vi "delete PID from configuration.vi"(8 "error in":errorcluster, 10 "PID Loop ID In":string, 11 "Tagbus PID Module configuration in":refnum<class "PID Module configuration.lvclass">) -> (0 "error out":errorcluster, 1 "index":i32, 2 "Deleted Loop":refnum<class "PID Loop.lvclass">, 3 "Tagbus PID Module configuration out":refnum<class "PID Module configuration.lvclass">)   [LabVIEW 2014, in "PID Module configuration.lvclass"]
doc: "This VI removes the specified VI from the Module Configuration."
uses:
  PID Module configuration.lvclass
  PID Loop.lvclass
  PID Module configuration.lvclass/PID Module configuration.ctl
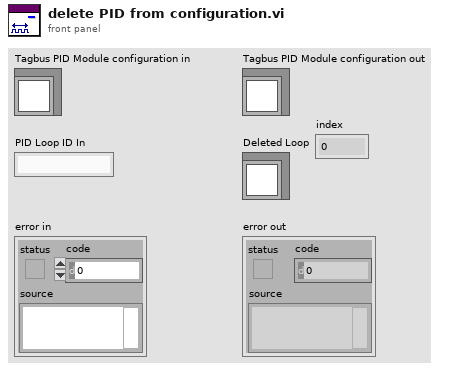
[diagram p1: front panel]
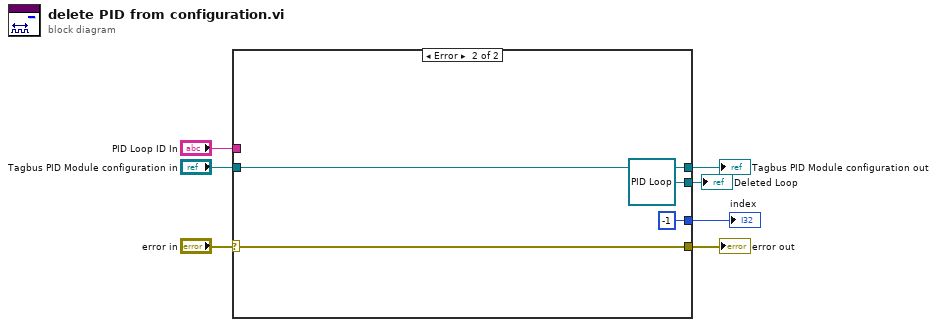
[diagram p0: block diagram]
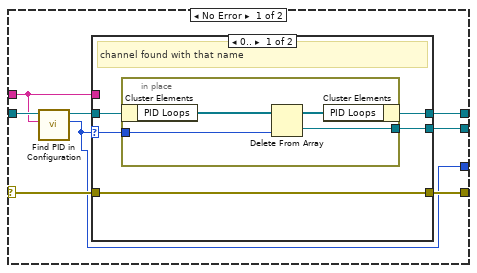
[diagram p2: hidden frame]
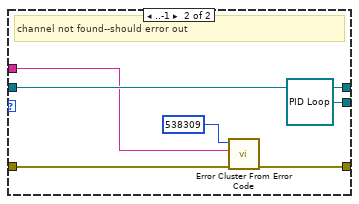
[diagram p3: hidden frame]
diagram:
  n1 = case shown="Error" "error in" {
    selector: "error in" -> [w11 w33]
    tunnel: "PID Loop ID In" -> [w10 _]
    tunnel: [w15 w33] -> w7
    tunnel: [w12 w34] -> w6
    tunnel: "Tagbus PID Module configuration in" -> [w14 w34]
    tunnel: [w9 refnum<class "PID Loop.lvclass"> refnum ("PID Loop.lvclass")] -> w2
    tunnel: [w8 -1 ("index")] -> w1
    frame No Error {
      n2 = call "Find PID in Configuration.vi"("PID Loop ID in"=w10, "Tagbus PID Module configuration in"=w14) -> ("index"=w8:i32, "Tagbus PID Module configuration out"=w13:refnum<class "PID Module configuration.lvclass">)  [unwired: 8 in]
      n3 = case shown="0.." w8 {
        selector: w8 -> [w20 _]
        tunnel: [w17 w30] -> w15
        tunnel: [w19 w28] -> w12
        tunnel: w13 -> [w18 w28]
        tunnel: w11 -> [w17 w27]
        tunnel: w10 -> [_ w26]
        tunnel: [w16 refnum<class "PID Loop.lvclass"> refnum ("PID Loop.lvclass")] -> w9
        frame 0.. {
          # "channel found with that name"
          n4 = in-place {
            in-place-border: w20 -> [w24]
            in-place-border: [w21] -> w16
            n5 = in-place-cluster #1(w18) -> ("PID Loops"=w22:refnum<class "PID Loop.lvclass">[])
            n6 = Delete From Array(array=w22, index=w24) -> (deleted portion=w21:refnum<class "PID Loop.lvclass">, array with subset deleted=w23:refnum<class "PID Loop.lvclass">[])  [unwired: 1 in]
            n7 = in-place-cluster #1("PID Loops"=w23) -> (w19:refnum<class "PID Module configuration.lvclass">)
          }
        }
        frame ..-1 {
          # "channel not found--should error out"
          n8 = call <vilib>:"Error Cluster From Error Code.vi"("error in (no error)"=w27, "error message (\"\")"=w26, "error code (0)"=538309) -> ("error out"=w30:errorcluster)  [unwired: 6 in]
        }
      }
    }
    frame Error {
    }
  }
  "error out" <- w7
  "Tagbus PID Module configuration out" <- w6
  "Deleted Loop" <- w2
  "index" <- w1
